vi "fgv_joystick-info_remote.vi"(7 "init":enum16{"enable", "init", "read", "write"}(ring), 8 "error in":errorcluster, 11 "joystick info-in":T2) -> (0 "error out":errorcluster, 1 "opval":T1, 2 "v_val":cluster{dbl, dbl} {"?" format="%.1f"; "?" format="%#.1f"}, 3 "joystick info-out":T2)   [LabVIEW 2019]
uses:
  Ctrl/joystick_opval.ctl
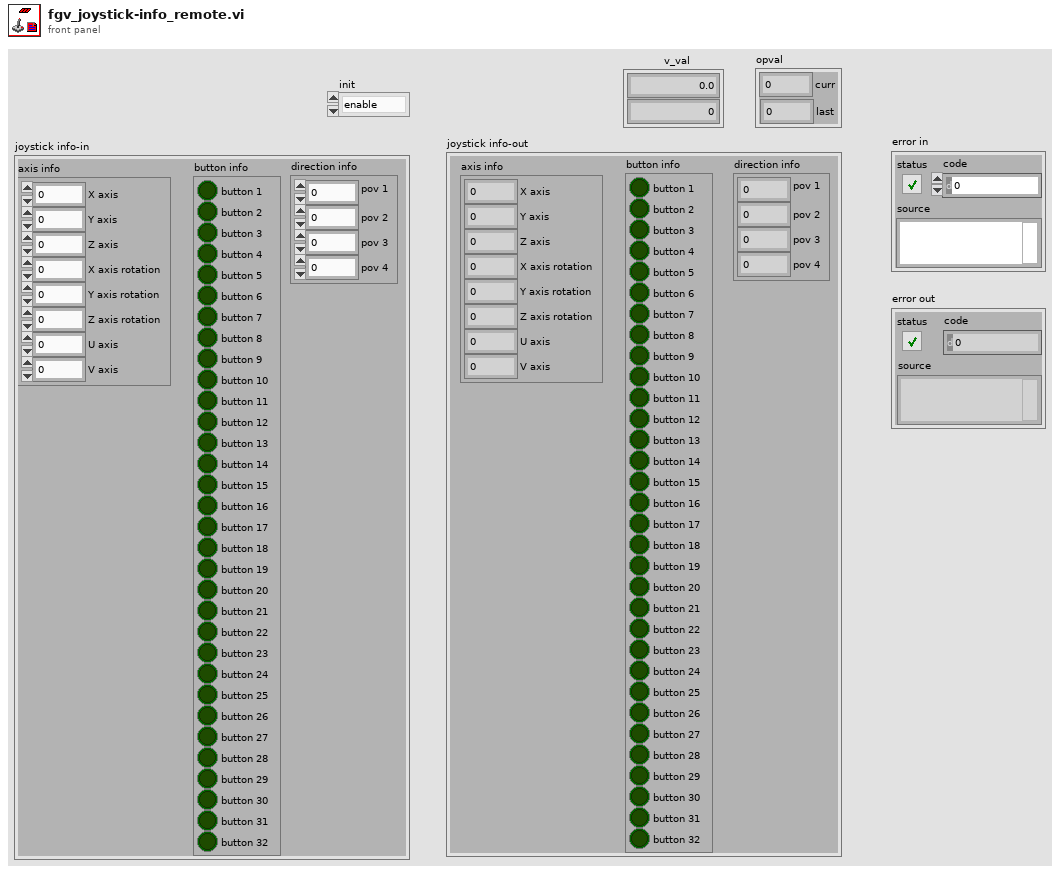
[diagram p1: front panel]
types:
  T1 = typedef "joystick_opval.ctl" = cluster{"curr":u32, "last":u32}
  T2 = cluster{"axis info":cluster{"X axis":i32, "Y axis":i32, "Z axis":i32, "X axis rotation":i32, "Y axis rotation":i32, "Z axis rotation":i32, "U axis":i32, "V axis":i32}, "button info":cluster{"button 1":bool, "button 2":bool, "button 3":bool, "button 4":bool, "button 5":bool, "button 6":bool, "button 7":bool, "button 8":bool, "button 9":bool, "button 10":bool, "button 11":bool, "button 12":bool, "button 13":bool, "button 14":bool, "button 15":bool, "button 16":bool, "button 17":bool, "button 18":bool, "button 19":bool, "button 20":bool, "button 21":bool, "button 22":bool, "button 23":bool, "button 24":bool, "button 25":bool, "button 26":bool, "button 27":bool, "button 28":bool, "button 29":bool, "button 30":bool, "button 31":bool, "button 32":bool}, "direction info":cluster{"pov 1":i32, "pov 2":i32, "pov 3":i32, "pov 4":i32}}
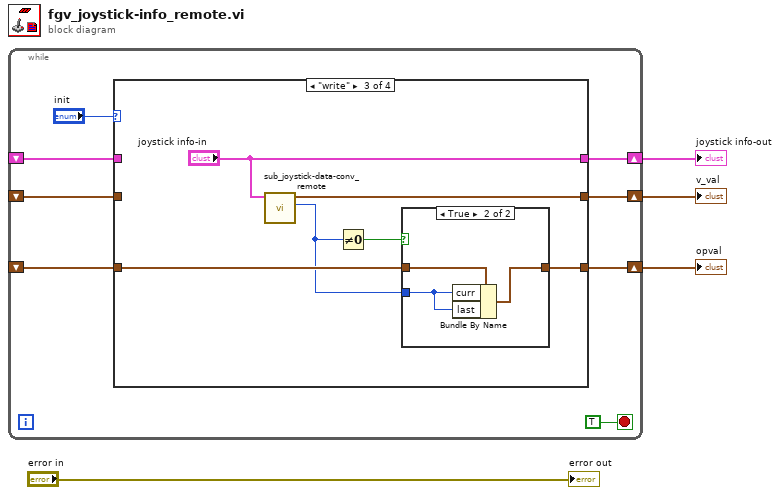
[diagram p0: block diagram]
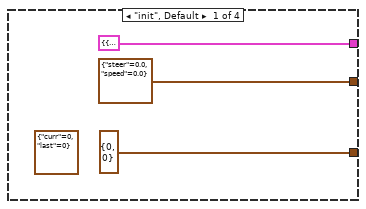
[diagram p2: hidden frame]
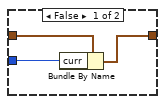
[diagram p4: hidden frame]
diagram:
  n1 = while {
    shift-right: [w10] -> w3
    shift-left: _ -> [w9]
    shift-right: [w7] -> w2
    shift-left: _ -> [w8]
    shift-right: [w6] -> w1
    shift-left: _ -> [w5]
    stop <- TRUE stop-if-true
    n2 = case shown="\"write\"" "init" {
      tunnel: [T2 {"axis info"={"X axis"=0, "Y axis"=0, "Z axis"=0, "X axis rotation"=0, "Y axis rotation"=0, "Z axis rotation"=0, "U axis"=0, "V axis"=0}, "button info"={"button 1"=FALSE, "button 2"=FALSE, "button 3"=FALSE, "button 4"=FALSE, "button 5"=FALSE, "button 6"=FALSE, "button 7"=FALSE, "button 8"=FALSE, "button 9"=FALSE, "button 10"=FALSE, "button 11"=FALSE, "button 12"=FALSE, "button 13"=FALSE, "button 14"=FALSE, "button 15"=FALSE, "button 16"=FALSE, "button 17"=FALSE, "button 18"=FALSE, "button 19"=FALSE, "button 20"=FALSE, "button 21"=FALSE, "button 22"=FALSE, "button 23"=FALSE, "button 24"=FALSE, "button 25"=FALSE, "button 26"=FALSE, "button 27"=FALSE, "button 28"=FALSE, "button 29"=FALSE, "button 30"=FALSE, "button 31"=FALSE, "button 32"=FALSE}, "direction info"={"pov 1"=0, "pov 2"=0, "pov 3"=0, "pov 4"=0}} ("joystick") w18 "joystick info-in" w33] -> w10
      tunnel: w9 -> [_ w18 _ w33]
      tunnel: [cluster{"steer":dbl, "speed":dbl} {"steer"=0.0, "speed"=0.0} ("Cluster") w17 w19 w32] -> w7
      tunnel: w8 -> [_ w17 _ w32]
      tunnel: [T1 {"curr"=0, "last"=0} ("opval") w16 w22 w31] -> w6
      tunnel: w5 -> [_ w16 w23 w31]
      frame "init", Default {
        (unwired) cluster{"curr":u32, "last":u32} {"curr"=0, "last"=0} ("opval")
      }
      frame "read" {
      }
      frame "write" {
        n3 = call "sub_joystick-data-conv_remote.vi"("joystick info-in"="joystick info-in") -> ("cmd"=w21:u32, "opval"=w19:cluster{dbl, dbl})  [unwired: 9 in]
        n4 = Not Equal To 0?(x=w21) -> (x != 0?=w24:bool)
        n5 = case shown="True" w24 {
          tunnel: w23 -> [w27 w30]
          tunnel: w21 -> [w26 w28]
          tunnel: [w25 w29] -> w22
          frame False {
            n6 = Bundle By Name(cluster=w27, "curr"=w26) -> (w25:T1)
          }
          frame True {
            n7 = Bundle By Name(cluster=w30, "curr"=w28, "last"=w28) -> (w29:T1)
          }
        }
      }
      frame "enable" {
      }
    }
  }
  "joystick info-out" <- w3
  "v_val" <- w2
  "opval" <- w1
  "error out" <- "error in"
